vi "Determine Warnings SubVI.vi"(5 "Max Wind Speed":dbl=10.0, 7 "Current Wind Speed":dbl, 8 "error in (no error)":errorcluster, 9 "Min Temp":dbl=10.0, 10 "Max Temp":dbl=30.0, 11 "Current Temp":dbl=25.0) -> (0 "error out":errorcluster, 1 "Warning?":bool, 2 "Warning Text":string)   [LabVIEW 2015]
doc: "This simple VI throws a warning if the Current temp input is greater than the max temp input or less than the min temp input. \n\nIt also throws a warning if the wind speed is above a maximum wind speed."
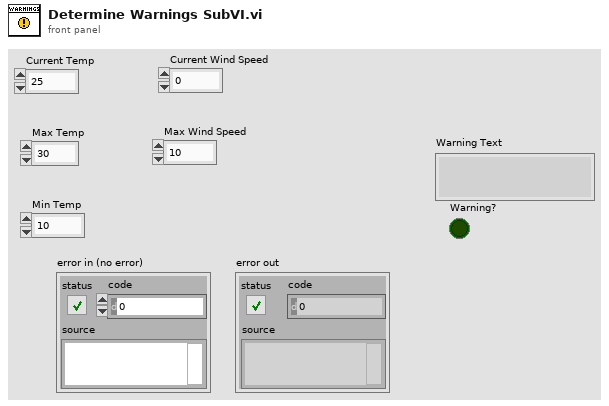
[diagram p1: front panel]
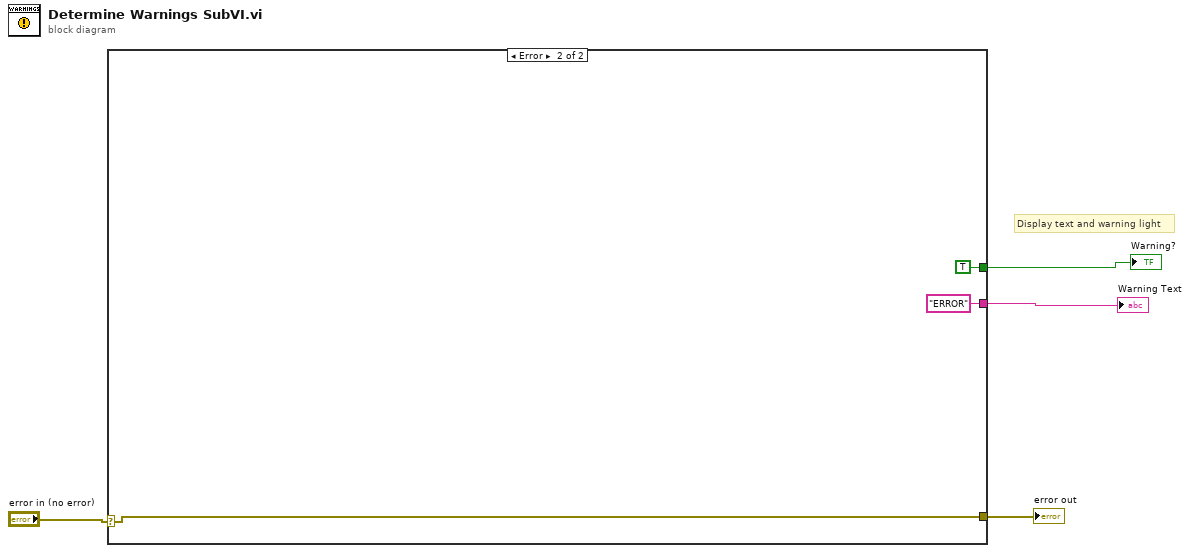
[diagram p0: block diagram]
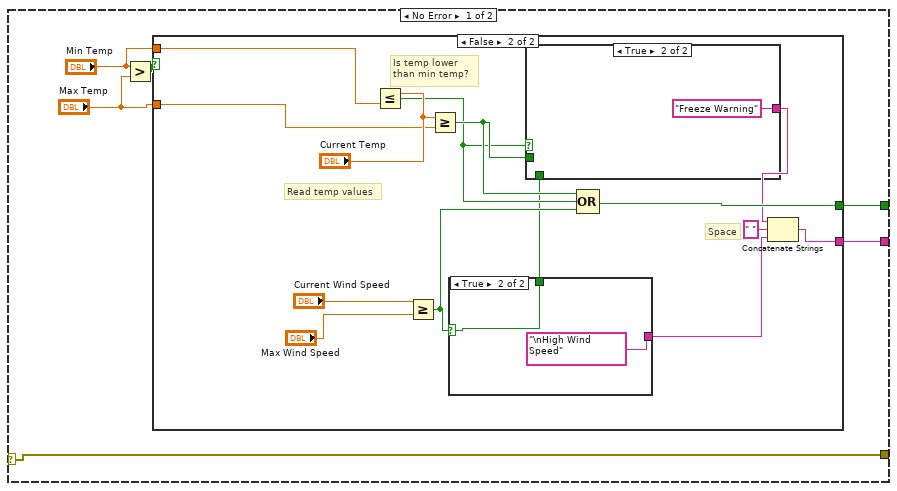
[diagram p2: hidden frame]
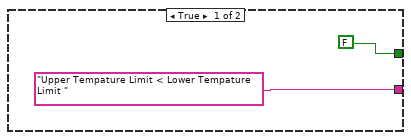
[diagram p3: hidden frame]
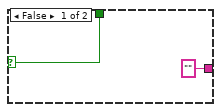
[diagram p4: hidden frame]
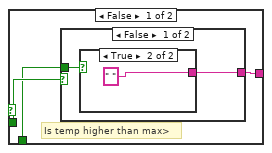
[diagram p5: hidden frame]
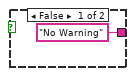
[diagram p6: hidden frame]
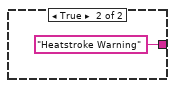
[diagram p7: hidden frame]
diagram:
  # "Display text and warning light"
  n1 = case shown="Error" "error in (no error)" {
    selector: "error in (no error)" -> [w5 w42]
    tunnel: [w10 TRUE] -> w4
    tunnel: [w6 "ERROR"] -> w3
    tunnel: [w5 w42] -> w1
    frame No Error {
      n2 = Greater?(x="Min Temp", y="Max Temp") -> (0:w9:bool)
      n3 = case shown="False" w9 {
        tunnel: "Max Temp" -> [_ w25]
        tunnel: "Min Temp" -> [_ w24]
        tunnel: [FALSE w23] -> w10
        tunnel: ["Upper Tempature Limit < Lower Tempature Limit " w16] -> w6
        frame True {
        }
        frame False {
          # "Space"
          # "Read temp values"
          # "Is temp lower \nthan min temp?"
          n4 = Less Or Equal?(x="Current Temp", y=w24) -> (x <= y?=w14:bool)
          n5 = Greater Or Equal?(x="Current Wind Speed", y="Max Wind Speed") -> (x >= y?=w20:bool)
          n6 = Greater Or Equal?(x="Current Temp", y=w25) -> (x >= y?=w15:bool)
          n7 = case shown="True" w20 {
            selector: w20 -> [w27 w29]
            tunnel: ["" "\nHigh Wind Speed"] -> w18
            tunnel: [w27 w29] -> w13
            frame False {
            }
            frame True {
            }
          }
          n8 = case shown="True" w14 {
            tunnel: [w32 "Freeze Warning"] -> w17
            tunnel: w15 -> [w33 _]
            tunnel: w13 -> [w31 _]
            frame False {
              # "Is temp higher than max>"
              n9 = case shown="False" w33 {
                tunnel: [w35 "Heatstroke Warning"] -> w32
                tunnel: w31 -> [w34 _]
                frame False {
                  n10 = case shown="True" w34 {
                    tunnel: ["No Warning" " "] -> w35
                    frame False {
                    }
                    frame True {
                    }
                  }
                }
                frame True {
                }
              }
            }
            frame True {
            }
          }
          n11 = Compound Arithmetic op=OR(w15, w14, w20) -> (w23:bool)
          n12 = Concatenate Strings(w17, " " ("string"), w18) -> (w16:string)
        }
      }
    }
    frame Error {
    }
  }
  "Warning Text" <- w3
  "Warning?" <- w4
  "error out" <- w1
